vi "Main.vi"() -> ()   [LabVIEW 2018]
doc: "Use this template to build a simple state machine design pattern. Each state executes code and determines which state to transition to."
uses:
  controls/State.ctl
  controls/Data.ctl
  controls/Configuration Settings.ctl
  controls/File Type.ctl
panel:
  in  "File Type":T1
  in  "Open File Location":bool
  in  "Open":bool
  in  "Save":bool
  out "Data":dbl[](graph)
  in  "Reset Settings":bool
  in  "Clear Graph":bool
  in  "Analyse  Data":bool
  in  "Acquire Data":bool
  in  "Configure Data":bool
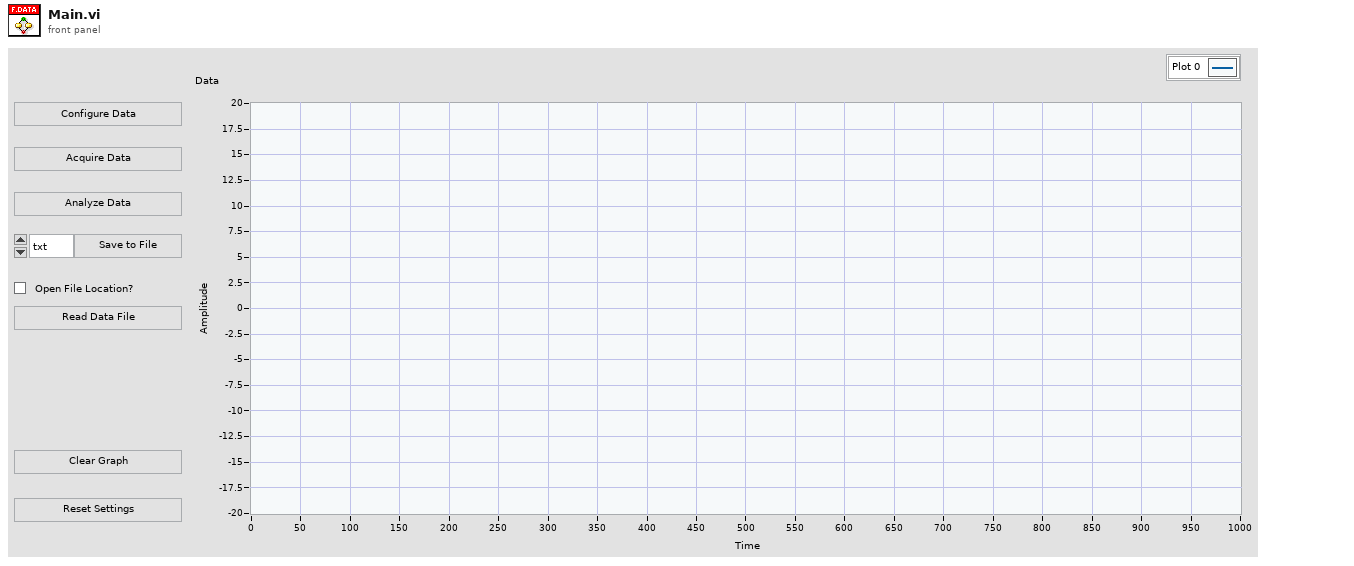
[diagram p1: front panel]
types:
  T1 = typedef "File Type.ctl" = enum16{"txt", "csv", "tdms"}
  T2 = typedef "Data.ctl" = cluster{"Configuration Settings":T3, "Data":dbl[]}
  T3 = typedef "Configuration Settings.ctl" = cluster{"Signal type":enum16{"Sine Wave", "Triangle Wave", "Square Wave", "Sawtooth Wave"}, "Amplitude":dbl, "Offset":dbl, "Amplitude 2":dbl, "Frequency":dbl}
  T4 = typedef "State.ctl" = enum16{"Initialize", "Wait for Event", "Configure", "Acquire Data State", "Update User Interface", "Reset Data", "Open Data File", "Save Data File", "Clear Data", "Analyse Data", "Stop", "Error"}
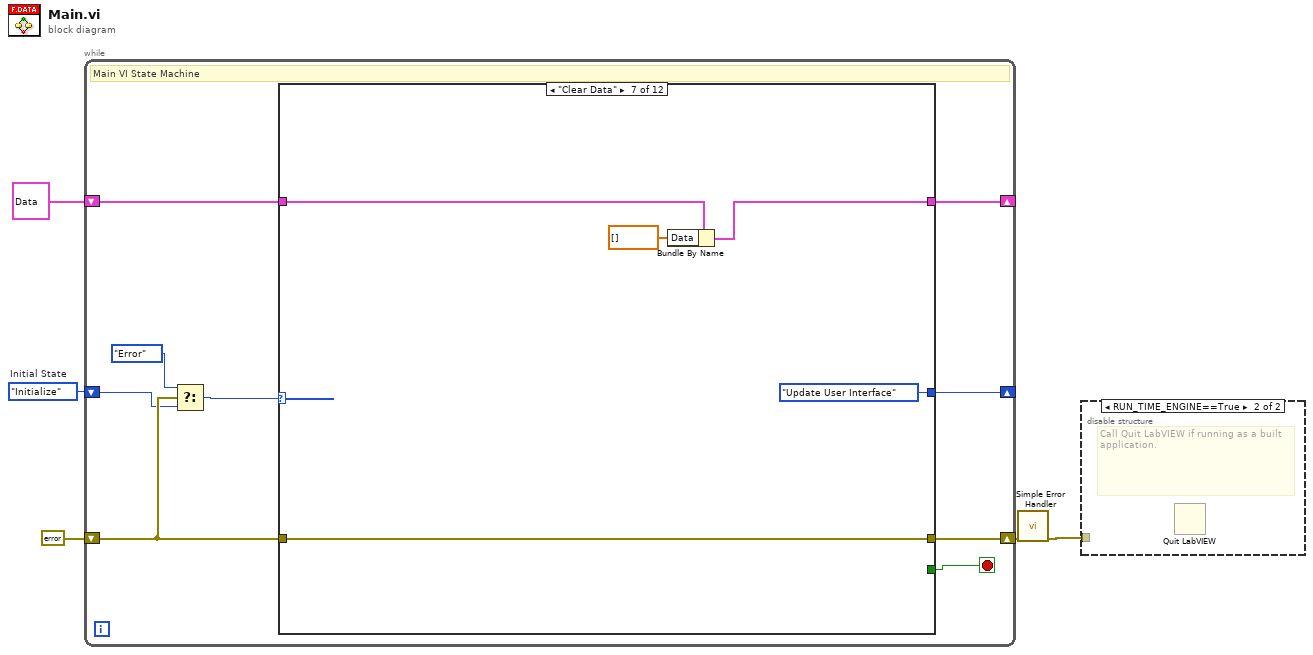
[diagram p0: block diagram]
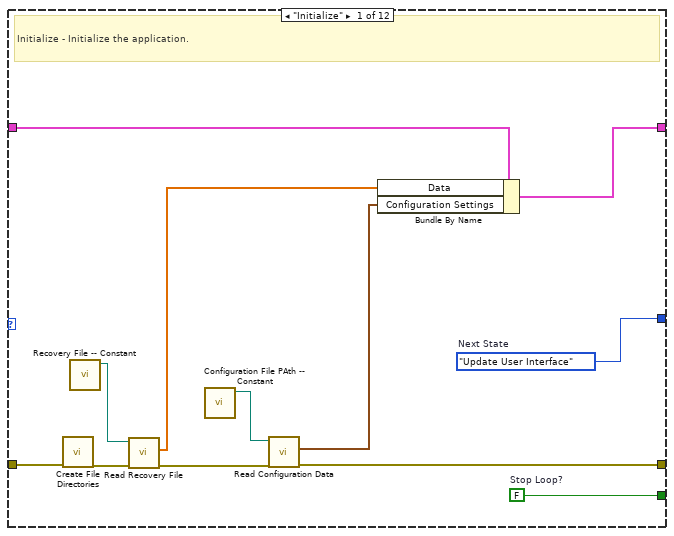
[diagram p3: hidden frame]
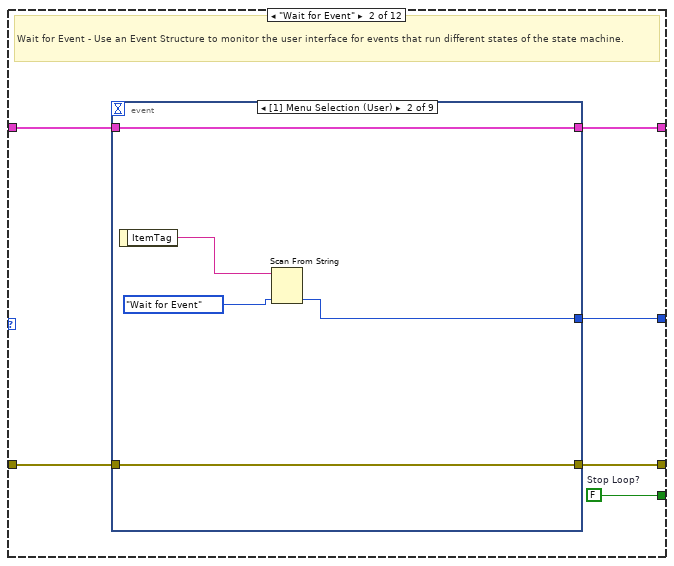
[diagram p4: hidden frame]
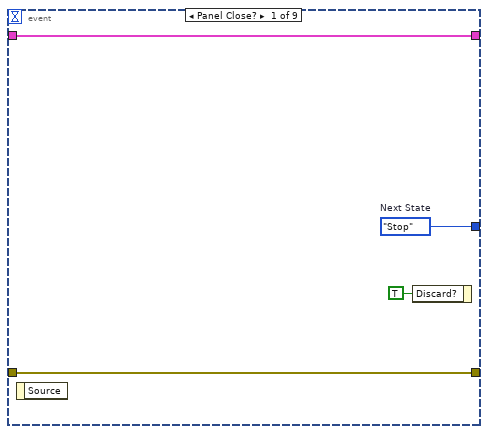
[diagram p5: hidden frame]
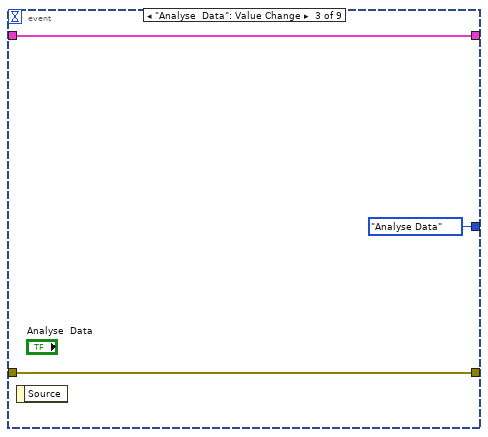
[diagram p6: hidden frame]
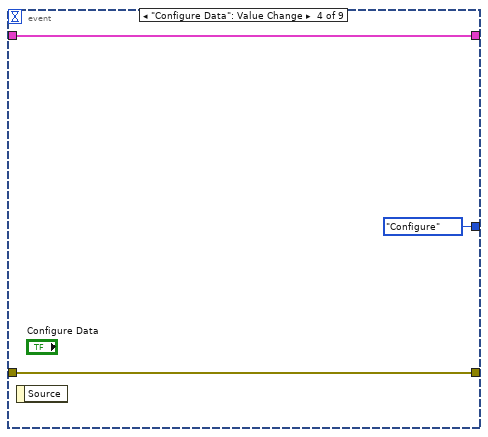
[diagram p7: hidden frame]
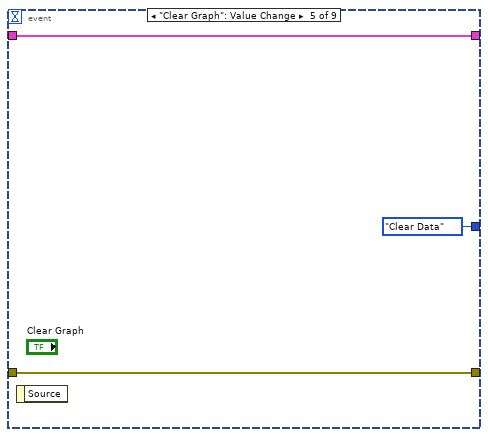
[diagram p8: hidden frame]
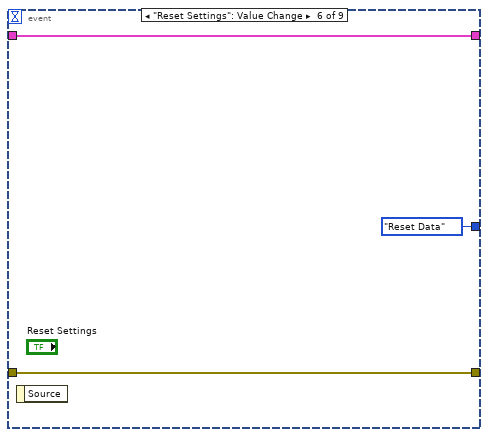
[diagram p9: hidden frame]
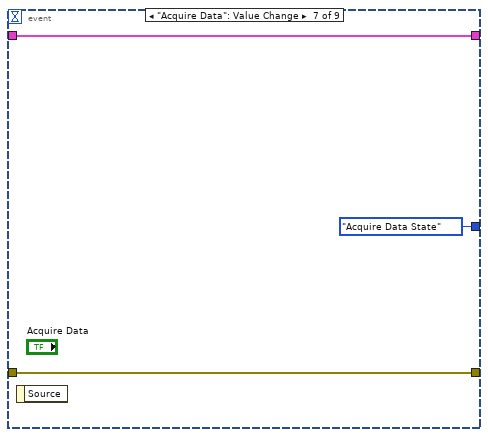
[diagram p10: hidden frame]
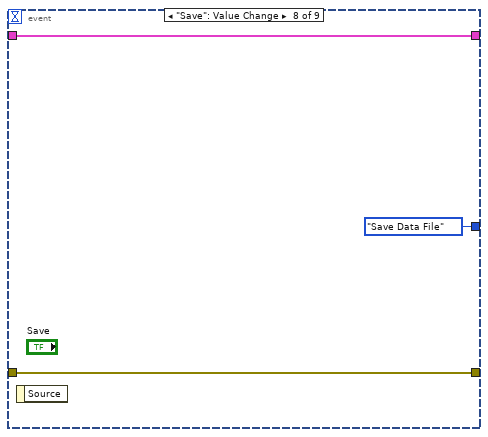
[diagram p11: hidden frame]
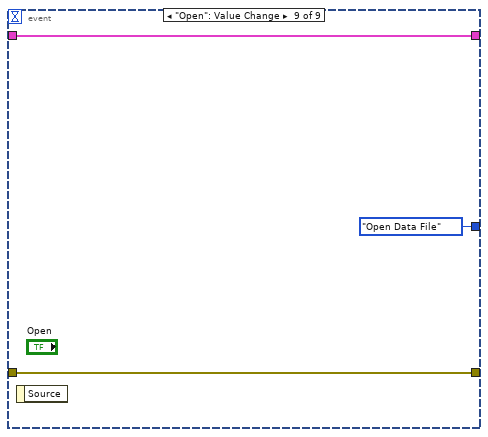
[diagram p12: hidden frame]
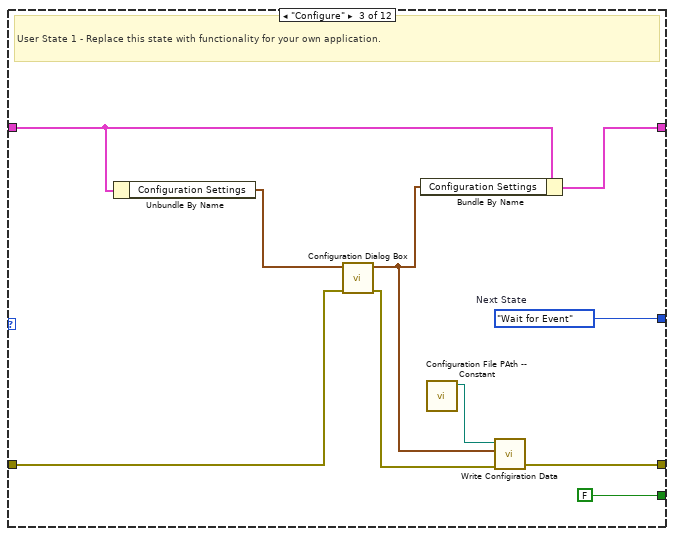
[diagram p13: hidden frame]
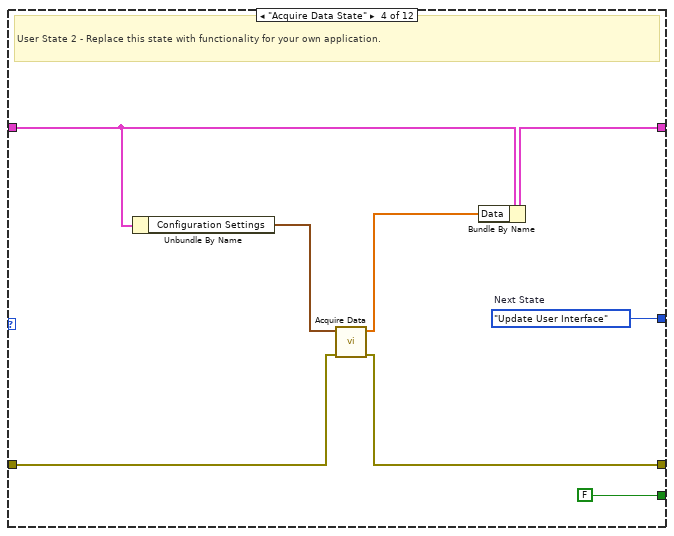
[diagram p14: hidden frame]
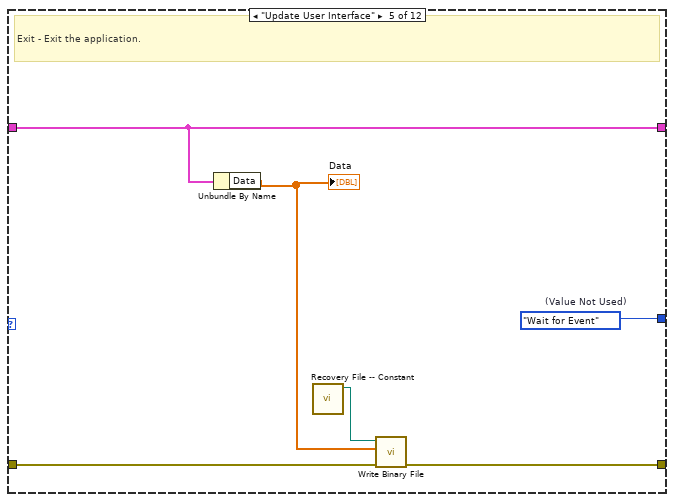
[diagram p15: hidden frame]
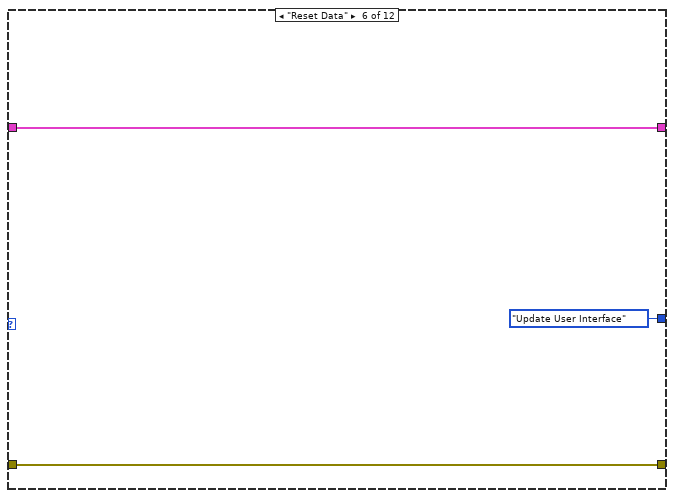
[diagram p16: hidden frame]
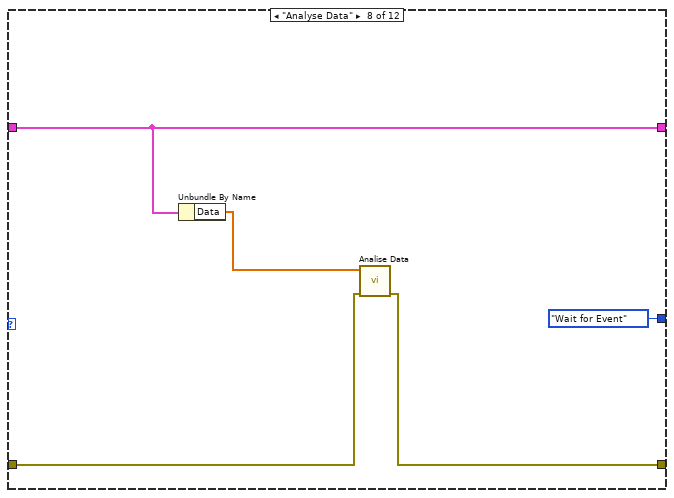
[diagram p17: hidden frame]
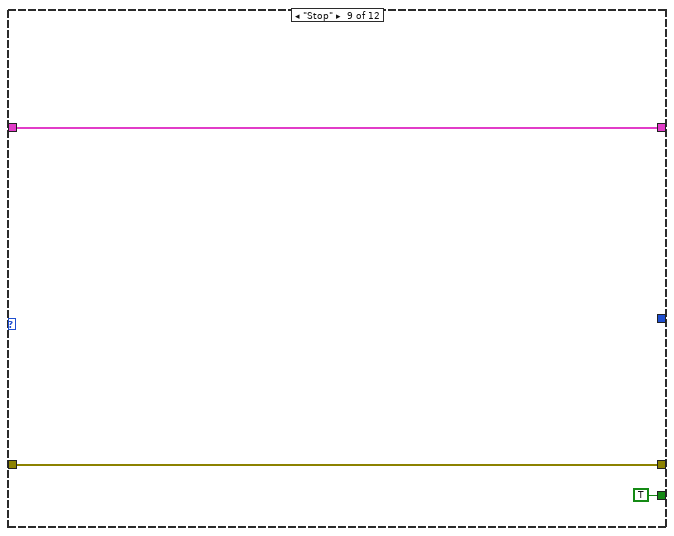
[diagram p18: hidden frame]
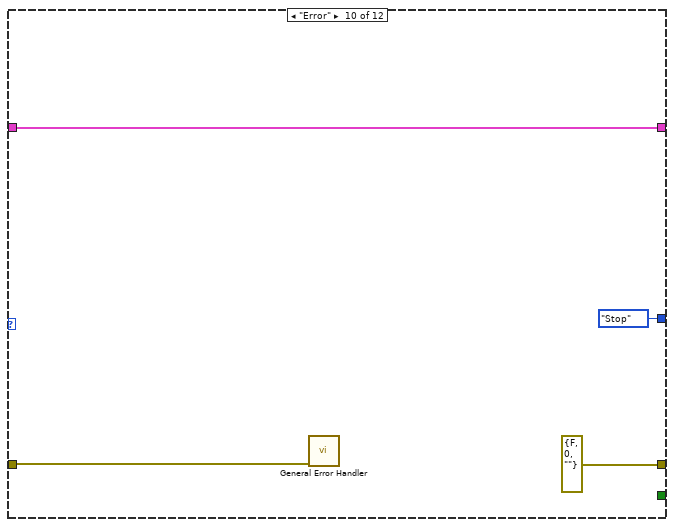
[diagram p19: hidden frame]
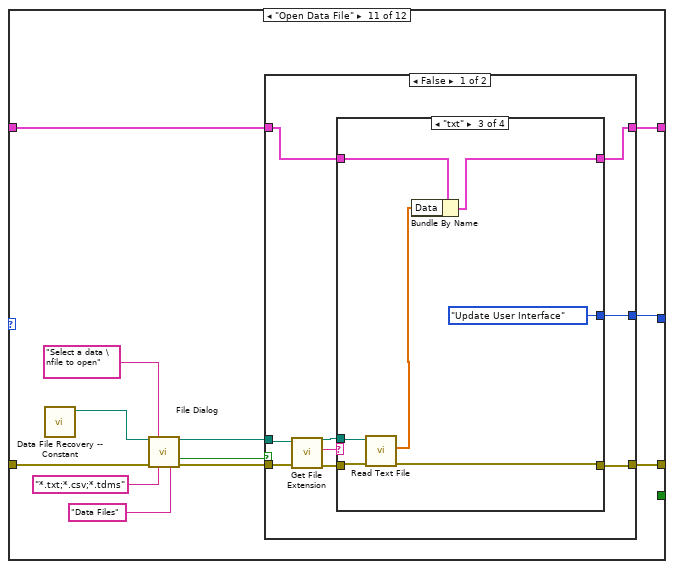
[diagram p20: hidden frame]
diagram:
  w5 = State."Initialize"  # Initial State
  n1 = while {
    shift-right: [w14] -> _
    shift-left: w5 -> [w8]
    shift-right: [w12] -> _
    shift-left: T2 {"Configuration Settings"={"Signal type"=enum."Sine Wave", "Amplitude"=1.0, "Offset"=0.0, "Amplitude 2"=1.0, "Frequency"=10.0}, "Data"=[]} ("Data") -> [w13]
    shift-right: [w11] -> w2
    shift-left: errorcluster {"status"=FALSE, "code"=0, "source"=""} ("error constant") -> [w10]
    stop <- w6 stop-if-true
    # "Main VI State Machine"
    n2 = Select(t=State."Error", s=w10, f=w8) -> (s? t:f=w9:T4)
    n3 = case shown="\"Clear Data\"" w9 {
      tunnel: [w26 w32 w72 w80 w86 State."Update User Interface" ("(Value Not Used)") State."Update User Interface" ("(Value Not Used)") State."Wait for Event" ("(Value Not Used)") _ State."Stop" ("(Value Not Used)") w111 State."Wait for Event" ("(Value Not Used)")] -> w14
      tunnel: [w25 w31 FALSE ("Stop Loop?") FALSE ("Stop Loop?") _ _ _ _ TRUE ("Stop Loop?") _ _ _] -> w6
      tunnel: w13 -> [w24 w30 w68 w74 w85 w89 w92 w96 w102 w106 w109 w163]
      tunnel: [w23 w29 w67 w73 w85 w89 w91 w96 w102 w106 w110 w163] -> w12
      tunnel: w10 -> [w19 w28 w70 w78 w83 w88 w94 w98 w101 w105 w118 w162]
      tunnel: [w22 w27 w65 w77 w84 w88 w94 w97 w101 errorcluster {"status"=FALSE, "code"=0, "source"=""} ("error constant") w115 w161] -> w11
      frame "Initialize" {
        w25 = FALSE  # Stop Loop?
        w26 = State."Update User Interface"  # Next State
        # "Initialize - Initialize the application."
        n4 = call "Create File Directories.vi"("error in (no error)"=w19) -> ("error out"=w17:errorcluster)  [unwired: 10 in]
        n5 = call "Recovery File -- Constant.vi"() -> ("Recovery File Path"=w15:path)  [unwired: 11 in]
        n6 = call "Read Recovery File.vi"("error in (no error)"=w17, "Path"=w15) -> ("error out"=w18:errorcluster, "Data Out"=w16:dbl[])  [unwired: 8 in]
        n7 = call "Configuration File PAth -- Constant.vi"() -> ("Configuration File Path"=w20:path)  [unwired: 11 in]
        n8 = call "Read Configuration Data.vi"("Path"=w20, "error in (no error)"=w18) -> ("Configuration Settings"=w21:T3, "error out"=w22:errorcluster)  [unwired: 7 in]
        n9 = Bundle By Name(cluster=w24, "Data"=w16, "Configuration Settings"=w21) -> (w23:T2)
      }
      frame "Wait for Event" {
        w31 = FALSE  # Stop Loop?
        # "Wait for Event - Use an Event Structure to monitor the user interface for events that run different states of the state machine."
        n10 = event shown="[1] Menu Selection (User)" {
          selector: _ -> [_ _ _ _ _ _ _ _ _]
          dyn-events: _ -> [_ _ _ _ _ _ _ _ _]
          timeout: _ -> [_ _ _ _ _ _ _ _ _]
          tunnel: [w36 w37 State."Analyse Data" ("Next State") State."Configure" ("Next State") State."Clear Data" ("Next State") State."Reset Data" ("Next State") State."Acquire Data State" ("Next State") State."Save Data File" ("Next State") State."Open Data File" ("Next State")] -> w32
          tunnel: w30 -> [w35 w41 w44 w47 w50 w53 w56 w59 w62]
          tunnel: [w35 w41 w44 w47 w50 w53 w56 w59 w62] -> w29
          tunnel: w28 -> [w34 w40 w43 w46 w49 w52 w55 w58 w61]
          tunnel: [w34 w40 w43 w46 w49 w52 w55 w58 w61] -> w27
          event Panel Close? {
            w36 = State."Stop"  # Next State
            n11 = event-data() -> ()  [unwired: 1 in, 1 out]
            n12 = event-data("Discard?"=TRUE) -> ()  [unwired: 1 in, 1 out]
          }
          event Menu Selection (User) {
            n13 = event-data() -> ("ItemTag"=w39:string)  [unwired: 1 in]
            n14 = Scan From String(input string=w39, default 1=State."Wait for Event" ("Next State")) -> (output 1=w37:T4)  [unwired: 3 in, 3 out]
          }
          event "Analyse  Data": Value Change {
            n15 = event-data() -> ()  [unwired: 1 in, 1 out]
          }
          event "Configure Data": Value Change {
            n16 = event-data() -> ()  [unwired: 1 in, 1 out]
          }
          event "Clear Graph": Value Change {
            n17 = event-data() -> ()  [unwired: 1 in, 1 out]
          }
          event "Reset Settings": Value Change {
            n18 = event-data() -> ()  [unwired: 1 in, 1 out]
          }
          event "Acquire Data": Value Change {
            n19 = event-data() -> ()  [unwired: 1 in, 1 out]
          }
          event "Save": Value Change {
            n20 = event-data() -> ()  [unwired: 1 in, 1 out]
          }
          event "Open": Value Change {
            n21 = event-data() -> ()  [unwired: 1 in, 1 out]
          }
        }
      }
      frame "Configure" {
        w72 = State."Wait for Event"  # Next State
        # "User State 1 - Replace this state with functionality for your own application."
        n22 = Unbundle By Name(w68) -> ("Configuration Settings"=w69:T3)
        n23 = call "Configuration Dialog Box.vi"("error in (no error)"=w70, "Configuration Settings In"=w69) -> ("error out"=w64:errorcluster, "Configuration Settings Out"=w66:T3)  [unwired: 8 in]
        n24 = Bundle By Name(cluster=w68, "Configuration Settings"=w66) -> (w67:T2)
        n25 = call "Configuration File PAth -- Constant.vi"() -> ("Configuration File Path"=w63:path)  [unwired: 11 in]
        n26 = call "Write Configiration Data.vi"("error in (no error)"=w64, "Configuration Settings"=w66, "Path"=w63) -> ("error out"=w65:errorcluster)  [unwired: 8 in]
      }
      frame "Acquire Data State" {
        w80 = State."Update User Interface"  # Next State
        # "User State 2 - Replace this state with functionality for your own application."
        n27 = Unbundle By Name(w74) -> ("Configuration Settings"=w76:T3)
        n28 = call "Acquire Data.vi"("error in (no error)"=w78, "Configuration Settings"=w76) -> ("error out"=w77:errorcluster, "Data Out"=w75:dbl[])  [unwired: 8 in]
        n29 = Bundle By Name(cluster=w74, "Data"=w75) -> (w73:T2)
      }
      frame "Update User Interface" {
        w86 = State."Wait for Event"  # (Value Not Used)
        # "Exit - Exit the application."
        n30 = Unbundle By Name(w85) -> ("Data"=w82:dbl[])
        "Data" <- w82
        n31 = call "Recovery File -- Constant.vi"() -> ("Recovery File Path"=w81:path)  [unwired: 11 in]
        n32 = call "Write Binary File.vi"("error in (no error)"=w83, "Data In"=w82, "Path"=w81) -> ("error out"=w84:errorcluster)  [unwired: 8 in]
      }
      frame "Reset Data" {
      }
      frame "Clear Data" {
        n33 = Bundle By Name(cluster=w92, "Data"=dbl[] []) -> (w91:T2)
      }
      frame "Analyse Data" {
        n34 = Unbundle By Name(w96) -> ("Data"=w95:dbl[])
        n35 = call "Analise Data.vi"("error in (no error)"=w98, "Data in"=w95) -> ("error out"=w97:errorcluster)  [unwired: 9 in]
      }
      frame "Stop" {
      }
      frame "Error" {
        n36 = call <vilib>:"General Error Handler.vi"("error in (no error)"=w105) -> ()  [unwired: 10 in, 5 out]
      }
      frame "Open Data File" {
        n37 = call "Data File Recovery -- Constant.vi"() -> ("Data File Directory"=w107:path)  [unwired: 11 in]
        n38 = call "File Dialog"("start path"=w107, "prompt"="Select a data \nfile to open", "error in"=w118, "pattern (all files)"="*.txt;*.csv;*.tdms" ("default name"), "pattern label"="Data Files") -> ("selected path"=w112:path, "cancelled"=w117:bool, "error out"=w116:errorcluster)  [unwired: 7 in, 1 out]
        n39 = case shown="False" w117 {
          tunnel: w116 -> [w127 w154]
          tunnel: [w124 w155] -> w115
          tunnel: w112 -> [w126 _]
          tunnel: [w120 State."Wait for Event" ("(Value Not Used)")] -> w111
          tunnel: [w121 w156] -> w110
          tunnel: w109 -> [w122 w156]
          frame False {
            n40 = call <vilib>:"Get File Extension.vi"("error in (no error)"=w127, "file"=w126) -> ("error out"=w125:errorcluster, "lowercase file extension"=w123:string, "dup file"=w119:path)  [unwired: 5 in, 2 out]
            n41 = case shown="\"txt\"" w123 {
              tunnel: [w129 w135 w144 w151] -> w124
              tunnel: w125 -> [w129 w136 w143 w152]
              tunnel: w122 -> [w131 w138 w141 w148]
              tunnel: [w131 w137 w140 w147] -> w121
              tunnel: [State."Wait for Event" ("(Value Not Used)") State."Update User Interface" ("(Value Not Used)") State."Update User Interface" ("(Value Not Used)") State."Update User Interface" ("(Value Not Used)")] -> w120
              tunnel: w119 -> [_ w133 w142 w150]
              frame Default {
                n42 = One Button Dialog(message="File tye not supported") -> ()  [unwired: 1 in, 1 out]
              }
              frame "tdms" {
                n43 = call "Read TDMS File.vi"("error in (no error)"=w136, "Path"=w133) -> ("error out"=w135:errorcluster, "Data"=w134:dbl[])  [unwired: 8 in]
                n44 = Bundle By Name(cluster=w138, "Data"=w134) -> (w137:T2)
              }
              frame "txt" {
                n45 = call "Read Text File.vi"("error in (no error)"=w143, "Path"=w142) -> ("error out"=w144:errorcluster, "Data"=w139:dbl[])  [unwired: 8 in]
                n46 = Bundle By Name(cluster=w141, "Data"=w139) -> (w140:T2)
              }
              frame "csv" {
                n47 = call "Read CSV File.vi"("error in (no error)"=w152, "Path"=w150) -> ("error out"=w151:errorcluster, "Data Out"=w146:dbl[])  [unwired: 8 in]
                n48 = Bundle By Name(cluster=w148, "Data"=w146) -> (w147:T2)
              }
            }
          }
          frame True {
            n49 = call <vilib>:"Clear Errors.vi"("error in (no error)"=w154, "specific error code to clear (0: all)"=43) -> ("error out"=w155:errorcluster)  [unwired: 4 in, 1 out]
          }
        }
      }
      frame "Save Data File" {
        n50 = Unbundle By Name(w163) -> ("Data"=w159:dbl[])
        n51 = call "Save Data File.vi"("File Type"="File Type", "Data"=w159, "Open File Location"="Open File Location", "error in (no error)"=w162) -> ("error out"=w161:errorcluster)  [unwired: 6 in]
      }
    }
  }
  n52 = call <vilib>:"Simple Error Handler.vi"("error in (no error)"=w2) -> ("error out"=w1:errorcluster)  [unwired: 4 in, 4 out]
  n53 = disable-structure shown="RUN_TIME_ENGINE==True" {
    disable-tunnel: w1 -> [_ _]
    frame condition #0 (active) {
    }
    frame condition #1 {
      # "Call Quit LabVIEW if running as a built application."
      n54 = Quit LabVIEW() -> ()  [unwired: 1 in]
    }
  }
